vi "Stop Points.vi"(8 "error in":errorcluster, 11 "Task Base in":refnum<class "Task Base.lvclass">) -> (0 "error out":errorcluster, 3 "Task Base out":refnum<class "Task Base.lvclass">)   [LabVIEW 2023, in "HAL GOOP4.lvlib" / "Task Base.lvclass"]
uses:
  Task Base.lvclass
  Task Base.lvclass/Task Base.ctl
  Measure and Stimulus Subsystems/Measure and Stimulus Subsystems.lvclass
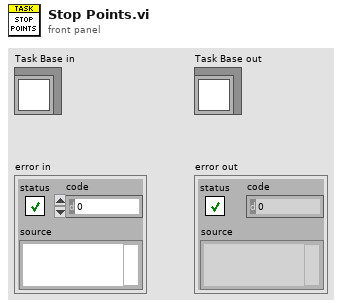
[diagram p1: front panel]
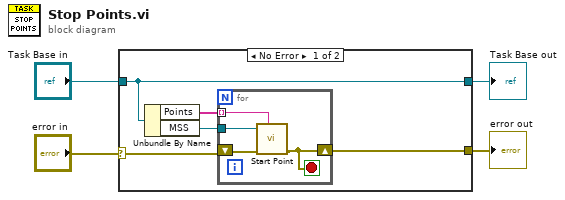
[diagram p0: block diagram]
diagram:
  n1 = case shown="No Error" "error in" {
    selector: "error in" -> [w9 w15]
    tunnel: [w5 w15] -> w3
    tunnel: [w6 w14] -> w1
    tunnel: "Task Base in" -> [w6 w14]
    frame No Error {
      n2 = Unbundle By Name(w6) -> ("Points"=w7:string[], "MSS"=w8:refnum<class "Measure and Stimulus Subsystems.lvclass">)
      n3 = for {
        tunnel: w8 -> [w13]
        shift-right: [w11] -> w5
        shift-left: w9 -> [w12]
        tunnel: w7 -> [w10] mode=indexing
        stop <- w11 stop-if-true
        n4 = call "Start Point.vi"("Point Ident"=w10, "error in"=w12, "MSS in"=w13) -> ("error out"=w11:errorcluster)  [unwired: 7 in, 1 out]
      }
    }
    frame Error {
    }
  }
  "error out" <- w3
  "Task Base out" <- w1
